vi "test_libssh2_session_timeout.vi"() -> ()   [LabVIEW 2013, in "libssh2_integration_tests.lvlib"]
uses:
  libssh2_integration_tests.lvlib
  <vilib>/addons/_JKI Toolkits/Caraya/classes/Test/Test.lvclass
  <vilib>/addons/_JKI Toolkits/Caraya/classes/Assert/Assert.lvclass
  libssh2/libssh2.lvlib
panel:
  out "error out":errorcluster
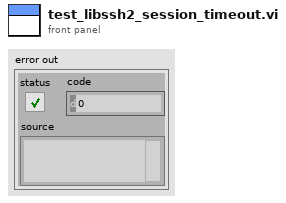
[diagram p1: front panel]
types:
  T1 = typedef "libssh2.lvlib/Session Refnum.ctl" = refnum<k1>
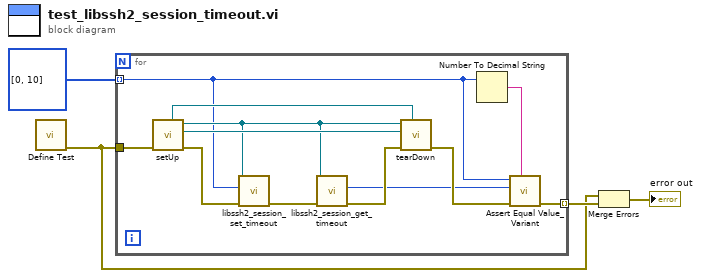
[diagram p0: block diagram]
diagram:
  n1 = call <vilib>:"Define Test.vi"() -> ("error out"=w2:errorcluster)  [unwired: 10 in, 1 out]
  n2 = for {
    tunnel: [w16] -> w4 mode=indexing
    tunnel: w2 -> [w15]
    tunnel: i32[] [0, 10] -> [w6] mode=indexing
    n3 = call "setUp.vi"("error in (no error)"=w15) -> ("error out"=w11:errorcluster, "connection ID"=w14:refnum<k5>, "session"=w8:T1, "fixture"=w13:refnum<class "Server Fixture.lvclass">)  [unwired: 7 in]
    n4 = call "libssh2_session_set_timeout.vi"("error in (no error)"=w11, "timeout in ms (0 = indefinite)"=w6, "session"=w8) -> ("error out"=w12:errorcluster)  [unwired: 8 in]
    n5 = call "libssh2_session_get_timeout.vi"("error in (no error)"=w12, "session"=w8) -> ("error out"=w9:errorcluster, "timeout in ms"=w7:i32)  [unwired: 8 in]
    n6 = call "tearDown.vi"("fixture"=w13, "error in (no error)"=w9, "connection ID"=w14, "session"=w8) -> ("error out"=w10:errorcluster)  [unwired: 7 in]
    n7 = Number To Decimal String(number=w6) -> (decimal integer string=w5:string)  [unwired: 1 in]
    n8 = call <vilib>:"Assert Equal Value_Variant.vi"("Label"=w5, "error in (no error)"=w10, "Y"=w7, "X"=w6) -> ("error out"=w16:errorcluster)  [unwired: 6 in, 1 out]
  }
  n9 = Merge Errors(w2, w4) -> (→"error out":errorcluster)
